vi "Seach config file.vi"(6 "working directory":path, 8 "extention":string=".json", 9 "pkg name":string="ms_teams") -> (0 "config file path":path, 3 "config file found?":bool)   [LabVIEW 2022 SP3]
uses:
  <vilib>/Utility/error.llb/Trim Whitespace One-Sided.vi
  <vilib>/Utility/sysdir.llb/System Directory Type.ctl
panel:
  # "The file location is chosen as follows\n\n1. $(working directory)/{pkg name}rc{extention}\n2. $HOME/.{pkg name}rc{extention}\n3. $HOME/.config/{pkg name}rc{extention}"
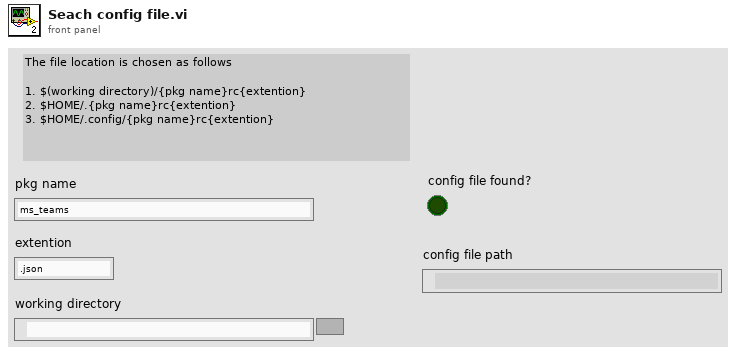
[diagram p1: front panel]
types:
  T1 = typedef "System Directory Type.ctl" = i32
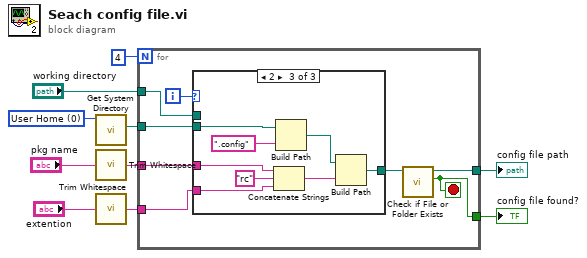
[diagram p0: block diagram]
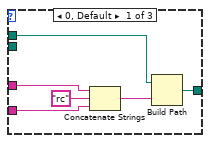
[diagram p2: hidden frame]
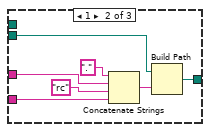
[diagram p3: hidden frame]
diagram:
  w2 = T1 0 items=["User Home"=0, "User Desktop"=1, "User Documents"=2, "User Application Data"=3, "User Preferences"=4, "User Temporary"=5, "Public Documents"=6, "Public Application Data"=7, "Public Preferences"=8, "Public Cache"=13, "System Core Libraries"=9, "System Installed Libraries"=10, "Application Files"=11, "Boot Volume Root"=12] ("system directory type")
  n1 = call <vilib>:"Get System Directory.vi"("system directory type"=w2) -> ("system directory"=w1:path)  [unwired: 10 in]
  n2 = call <vilib>:"Trim Whitespace.vi"("string"="pkg name") -> ("trimmed string"=w6:string)  [unwired: 1 in]
  n3 = call <vilib>:"Trim Whitespace.vi"("string"="extention") -> ("trimmed string"=w5:string)  [unwired: 1 in]
  n4 = for {
    N: 4 -> [_]
    tunnel: w6 -> [w17]
    tunnel: w5 -> [w16]
    tunnel: "working directory" -> [w15]
    tunnel: [w12] -> w3
    tunnel: w1 -> [w14]
    tunnel: [w11] -> w4
    i -> [w18]
    stop <- w11 stop-if-true
    n5 = case shown="2" w18 {
      tunnel: w17 -> [w23 w28 w38]
      tunnel: w16 -> [w22 w27 w37]
      tunnel: w15 -> [w20 _ _]
      tunnel: [w19 w26 w36] -> w13
      tunnel: w14 -> [_ w25 w35]
      frame 0, Default {
        n6 = Concatenate Strings(w23, "rc" ("string"), w22) -> (w21:string)
        n7 = Build Path(base path=w20, name or relative path=w21) -> (appended path=w19:path)
      }
      frame 1 {
        n8 = Concatenate Strings("." ("string"), w28, "rc" ("string"), w27) -> (w31:string)
        n9 = Build Path(base path=w25, name or relative path=w31) -> (appended path=w26:path)
      }
      frame 2 {
        n10 = Concatenate Strings(w38, "rc" ("string"), w37) -> (w32:string)
        n11 = Build Path(base path=w35, name or relative path=".config" ("string")) -> (appended path=w33:path)
        n12 = Build Path(base path=w33, name or relative path=w32) -> (appended path=w36:path)
      }
    }
    n13 = call <vilib>:"Check if File or Folder Exists.vi"("path"=w13) -> ("file or folder exists?"=w11:bool, "dup path"=w12:path)  [unwired: 8 in, 1 out]
  }
  "config file found?" <- w4
  "config file path" <- w3
